vi "Names Data Set.vi"(0 "Name Actions":T1, 11 "error in (no error)":errorcluster) -> (1 "Actuator Command Volts":string[](array[string])=["Command  X1 (V)", "Command  X2 (V)", "Command  Y1 (V)", "Command  Z1 (V)", "Command  Z2 (V)", "Command  Z3 (V)"], 2 "Actuator Volt Readings":string[](array[string])=["LVDT X1 (V)", "LVDT X2 (V)", "LVDT Y1 (V)", "LVDT Z1 (V)", "LVDT Z2 (V)", "LVDT Z3 (V)", "Load Cell X1 (V)", "Load Cell X2 (V)", "Load Cell Y1 (V)", "Load Cell Z1 (V)", "Load Cell Z2 (V)", "Load Cell Z3 (V)"], 3 "Servo Names":string[](array[string])=["Servo Error X1 (V)", "Servo Error X2 (V)", "Servo Error Y1 (V)", "Servo Error Z1 (V)", "Servo Error Z2 (V)", "Servo Error Z3 (V)"], 4 "Cartesian Commands":string[](array[string])=["CommandDx (in)", "CommandDy (in)", "CommandDz (in)", "CommandRx (rad)", "CommandRy (rad)", "CommandRz (rad)"], 6 "Cartesian Readings":string[](array[string])=["Dx (in)", "Dy (in)", "Dz (in)", "Rx (rad)", "Ry (rad)", "Rz (rad)", " Fx (lbs)", " Fy (lbs)", " Fz (lbs)", " Mx (lb*in)", " My (lb*in)", " Mz (lb*in)"], 8 "Actuator Commands":string[](array[string])=["Command  X1 (in)", "Command  X2 (in)", "Command  Y1 (in)", "Command  Z1 (in)", "Command  Z2 (in)", "Command  Z3 (in)"], 10 "Actuator Readings":string[](array[string])=["LVDT X1 (in)", "LVDT X2 (in)", "LVDT Y1 (in)", "LVDT Z1 (in)", "LVDT Z2 (in)", "LVDT Z3 (in)", "Load Cell X1 (lbs)", "Load Cell X2 (lbs)", "Load Cell Y1 (lbs)", "Load Cell Z1 (lbs)", "Load Cell Z2 (lbs)", "Load Cell Z3 (lbs)"], 13 "External Sensor Names":string[](array[string]), 14 "Cartesian Force Commands":string[](array[string])=["Command Fx (lbs)", "Command Fy (lbs)", "Command Fz (lbs)", "Command Mx (lb*in)", "Command My (lb*in)", "Command Mz (lb*in)"], 15 "error out":errorcluster)   [LabVIEW 2013]
uses:
  Name Actions.ctl
  Data Access Objects/Metadata/Persistant DAO Actions.ctl
  Apps/Unit Label Type.ctl
  Data Access Objects/Sensors/Sensor List Class.lvclass
panel:
  in  "Actuators":string[](array[string])=["X1", "X2", "Y1", "Z1", "Z2", "Z3"]
  in  "Cartesian Force":string[](array[string])=["Fx (lbs)", "Fy (lbs)", "Fz (lbs)", "Mx (lb*in)", "My (lb*in)", "Mz (lb*in)"]
  in  "Cartesian Displacement Units":string[](array[string])=["Dx (in)", "Dy (in)", "Dz (in)", "Rx (rad)", "Ry (rad)", "Rz (rad)"]
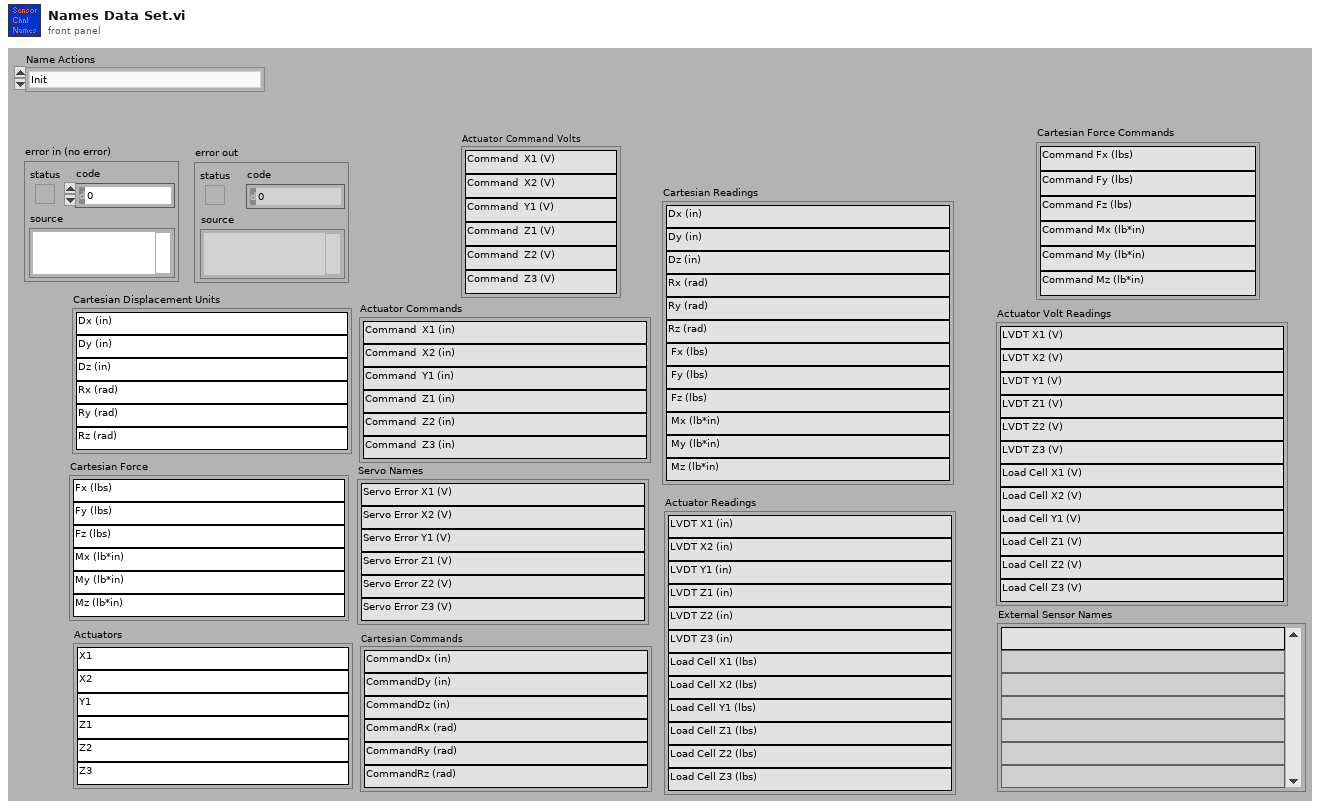
[diagram p1: front panel]
types:
  T1 = typedef "Name Actions.ctl" = enum16{"Init", "Get Names", "Get Index"}
  T2 = typedef "Unit Label Type.ctl" = enum16{"Actuator Displacement", "Actuator Force", "Cartesian Force", "Cartesian Translation", "Cartesian Rotation", "Cartesian Moment"}
  T3 = typedef "Persistant DAO Actions.ctl" = enum16{"Init", "Get", "Set", "Load", "Save"}
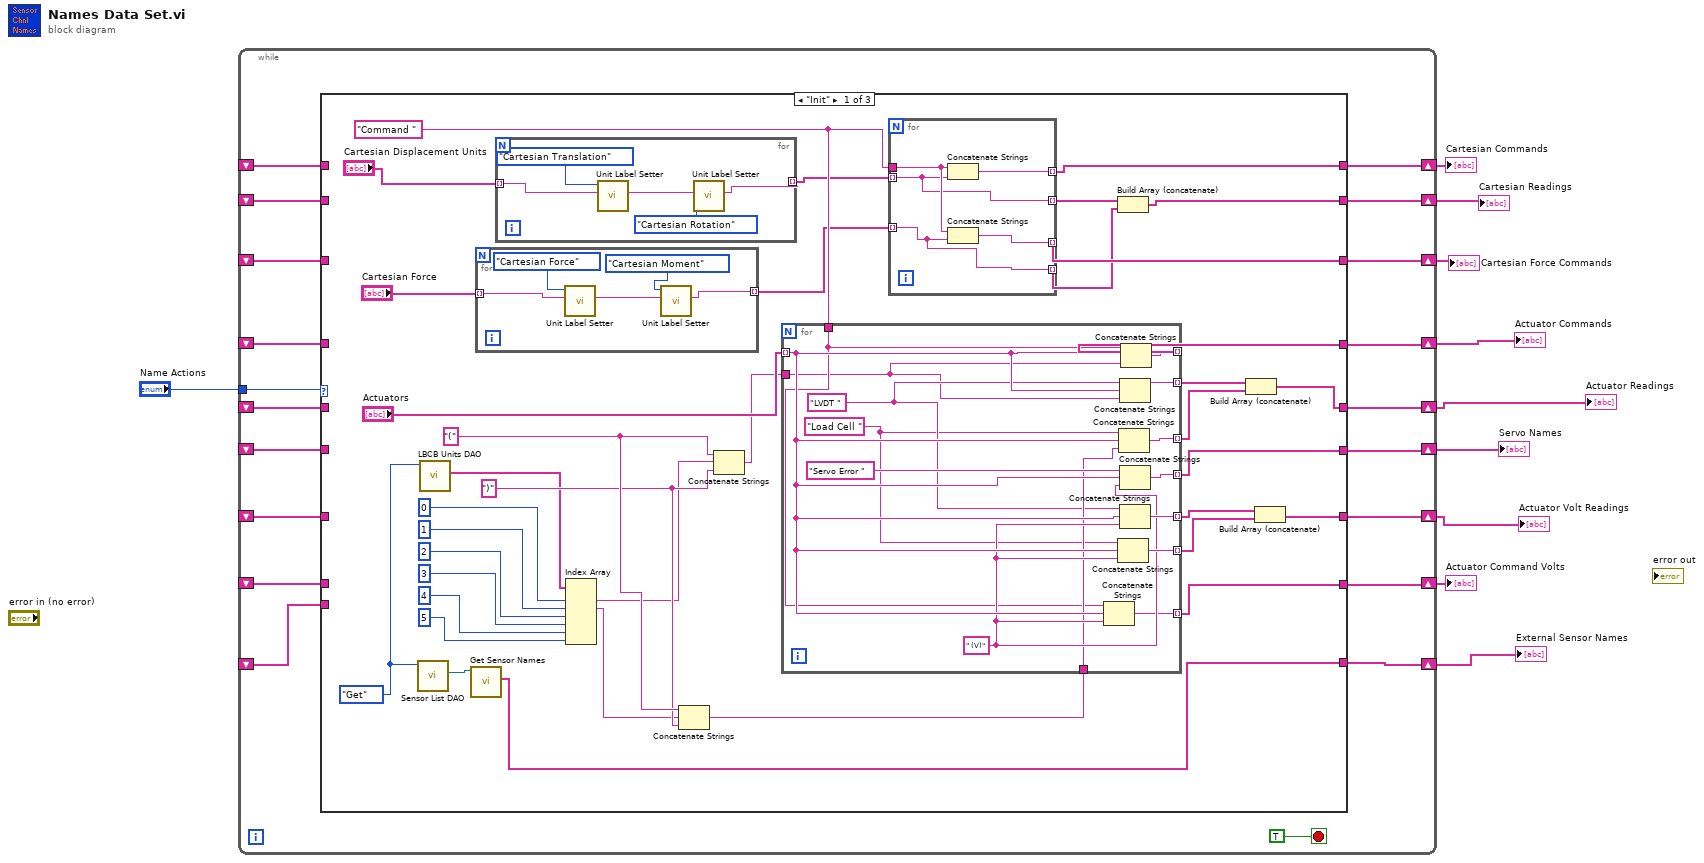
[diagram p0: block diagram]
diagram:
  n1 = while {
    tunnel: "Name Actions" -> [w29]
    shift-right: [w28] -> w9
    shift-left: _ -> [w24]
    shift-right: [w27] -> w8
    shift-left: _ -> [w22]
    shift-right: [w26] -> w7
    shift-left: _ -> [w23]
    shift-right: [w25] -> w6
    shift-left: _ -> [w21]
    shift-right: [w20] -> w5
    shift-left: _ -> [w19]
    shift-right: [w18] -> w4
    shift-left: _ -> [w17]
    shift-right: [w16] -> w3
    shift-left: _ -> [w15]
    shift-right: [w14] -> w2
    shift-left: _ -> [w13]
    shift-right: [w12] -> w1
    shift-left: _ -> [w11]
    stop <- TRUE stop-if-true
    n2 = case shown="\"Init\"" w29 {
      tunnel: [w60 w105 w114] -> w28
      tunnel: [w55 w103 w112] -> w27
      tunnel: [w54 w104 w113] -> w26
      tunnel: [w31 w102 w111] -> w25
      tunnel: w24 -> [_ w105 w114]
      tunnel: w23 -> [_ w104 w113]
      tunnel: w22 -> [_ w103 w112]
      tunnel: w21 -> [_ w102 w111]
      tunnel: [w59 w101 w110] -> w20
      tunnel: w19 -> [_ w101 w110]
      tunnel: [w57 w100 w109] -> w18
      tunnel: w17 -> [_ w100 w109]
      tunnel: [w58 w99 w108] -> w16
      tunnel: w15 -> [_ w99 w108]
      tunnel: [w56 w98 w107] -> w14
      tunnel: w13 -> [_ w98 w107]
      tunnel: [w53 w97 w106] -> w12
      tunnel: w11 -> [_ w97 w106]
      frame "Init" {
        w44 = ")" ("string")
        w45 = "(" ("string")
        w33 = Persistant_DAO_Actions."Get" ("Persistent DAO Actions")
        w51 = "Command " ("string")
        n3 = call "Sensor List DAO.vi"("Actions"=w33) -> ("Sensor List Out"=w32:refnum<class "Sensor List Class.lvclass">)  [unwired: 8 in, 2 out]
        n4 = call "LBCB Units DAO.vi"("Persistent DAO Actions"=w33) -> ("Unit Labels Out"=w42:string[])  [unwired: 6 in, 4 out]
        n5 = call "Get Sensor Names.vi"("Sensor List Class in"=w32) -> ("Names"=w31:string[])  [unwired: 8 in, 2 out]
        n6 = for {
          tunnel: "Cartesian Force" -> [w71] mode=indexing
          tunnel: [w69] -> w46 mode=indexing
          n7 = call "Unit Label Setter.vi"("Input String"=w71, "Label Type"=Unit_Label_Type."Cartesian Force") -> ("Output String"=w70:string)  [unwired: 9 in]
          n8 = call "Unit Label Setter.vi"("Input String"=w70, "Label Type"=Unit_Label_Type."Cartesian Moment") -> ("Output String"=w69:string)  [unwired: 9 in]
        }
        n9 = for {
          tunnel: "Cartesian Displacement Units" -> [w73] mode=indexing
          tunnel: [w72] -> w48 mode=indexing
          n10 = call "Unit Label Setter.vi"("Input String"=w73, "Label Type"=Unit_Label_Type."Cartesian Translation") -> ("Output String"=w74:string)  [unwired: 9 in]
          n11 = call "Unit Label Setter.vi"("Input String"=w74, "Label Type"=Unit_Label_Type."Cartesian Rotation") -> ("Output String"=w72:string)  [unwired: 9 in]
        }
        n12 = Index Array(array=w42, index #1=0 ("index"), index #2=1 ("index"), index #3=2 ("index"), index #4=3 ("index"), index #5=4 ("index"), index #6=5 ("index")) -> (element #1=w34:string, element #2=w35:string)  [unwired: 4 out]
        n13 = Concatenate Strings(w45, w35, w44) -> (w50:string)
        n14 = Concatenate Strings(w45, w34, w44) -> (w43:string)
        n15 = for {
          tunnel: "Actuators" -> [w84] mode=indexing
          tunnel: [w90] -> w57 mode=indexing
          tunnel: [w89] -> w64 mode=indexing
          tunnel: [w88] -> w63 mode=indexing
          tunnel: [w87] -> w54 mode=indexing
          tunnel: [w86] -> w62 mode=indexing
          tunnel: [w85] -> w61 mode=indexing
          tunnel: [w82] -> w56 mode=indexing
          tunnel: w50 -> [w81]
          tunnel: w51 -> [w78]
          tunnel: w43 -> [w77]
          w79 = "Load Cell " ("string")
          w80 = "LVDT " ("string")
          w83 = " (V)" ("string")
          n16 = Concatenate Strings(w78, w84, w83) -> (w82:string)
          n17 = Concatenate Strings(w79, w84, w83) -> (w85:string)
          n18 = Concatenate Strings(w79, w84, w81) -> (w88:string)
          n19 = Concatenate Strings(w80, w84, w77) -> (w89:string)
          n20 = Concatenate Strings("Servo Error " ("string"), w84, w83) -> (w87:string)
          n21 = Concatenate Strings(w80, w84, w83) -> (w86:string)
          n22 = Concatenate Strings(w78, w84, w77) -> (w90:string)
        }
        n23 = for {
          tunnel: w51 -> [w95]
          tunnel: w48 -> [w93] mode=indexing
          tunnel: [w96] -> w58 mode=indexing
          tunnel: [w93] -> w66 mode=indexing
          tunnel: w46 -> [w92] mode=indexing
          tunnel: [w94] -> w53 mode=indexing
          tunnel: [w92] -> w52 mode=indexing
          n24 = Concatenate Strings(w95, w93) -> (w96:string)
          n25 = Concatenate Strings(w95, w92) -> (w94:string)
        }
        n26 = Build Array (concatenate)(w66, w52) -> (w60:string[])
        n27 = Build Array (concatenate)(w64, w63) -> (w59:string[])
        n28 = Build Array (concatenate)(w62, w61) -> (w55:string[])
      }
      frame "Get Names" {
      }
      frame "Get Index" {
      }
    }
  }
  "Cartesian Readings" <- w9
  "Actuator Volt Readings" <- w8
  "Servo Names" <- w7
  "External Sensor Names" <- w6
  "Actuator Readings" <- w5
  "Actuator Commands" <- w4
  "Cartesian Commands" <- w3
  "Actuator Command Volts" <- w2
  "Cartesian Force Commands" <- w1
